vi "Get Ctl Value.vi"(8 "error in (no error)":errorcluster, 11 "Ring Field in":refnum<class "Ring Field.lvclass">) -> (0 "error out":errorcluster, 2 "Value":string, 3 "Ring Field out":refnum<class "Ring Field.lvclass">)   [LabVIEW 2020, in "Basic Fields.lvlib" / "Ring Field.lvclass"]
uses:
  Ring Field.lvclass
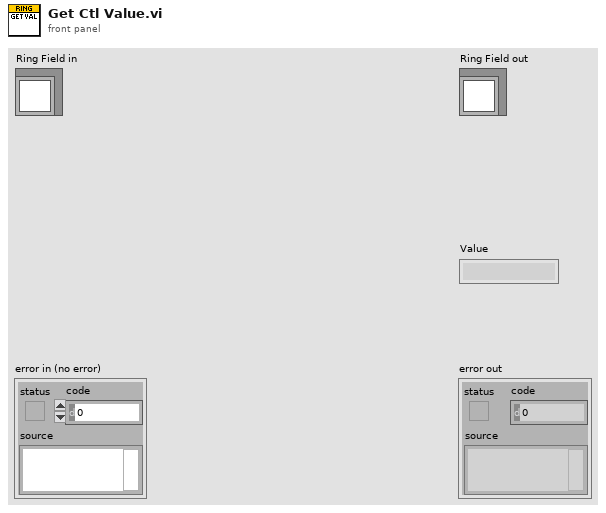
[diagram p1: front panel]
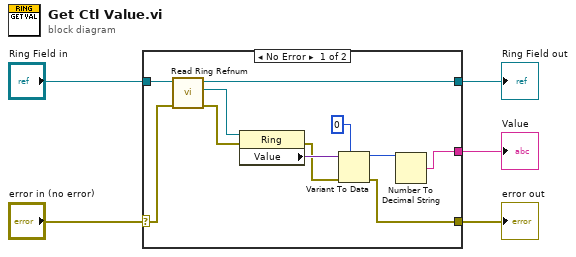
[diagram p0: block diagram]
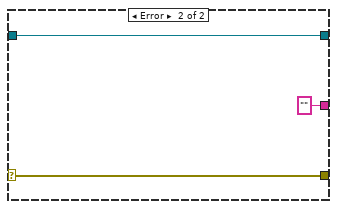
[diagram p2: hidden frame]
diagram:
  n1 = case shown="No Error" "error in (no error)" {
    selector: "error in (no error)" -> [w14 w18]
    tunnel: "Ring Field in" -> [w16 w19]
    tunnel: [w15 w19] -> w3
    tunnel: [w6 w18] -> w2
    tunnel: [w9 ""] -> w1
    frame No Error {
      n2 = call "Read Ring Refnum.vi"("error in (no error)"=w14, "Ring Field in"=w16) -> ("error out"=w8:errorcluster, "Ring Refnum"=w13:refnum<vi>, "Ring Field out"=w15:refnum<class "Ring Field.lvclass">)  [unwired: 7 in]
      n3 = property class="Ring"(reference=w13, error in=w8) -> (error out=w7:errorcluster, "Value"=w12:variant)  [unwired: 1 out]
      n4 = Variant To Data(error in=w7, type=0, Variant=w12) -> (data=w10:i32, error out=w6:errorcluster)
      n5 = Number To Decimal String(number=w10) -> (decimal integer string=w9:string)  [unwired: 1 in]
    }
    frame Error {
    }
  }
  "error out" <- w2
  "Ring Field out" <- w3
  "Value" <- w1
